vi "parse_speed.vi"(11 "Up Speed(mm/min)":dbl) -> (3 "String":string)   [LabVIEW 2017]
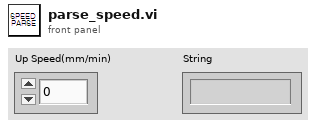
[diagram p1: front panel]
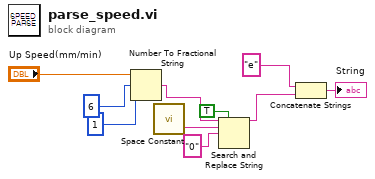
[diagram p0: block diagram]
diagram:
  n1 = Number To Fractional String(number="Up Speed(mm/min)", width (-)=6, precision (6)=1) -> (F-format string=w6:string)  [unwired: 1 in]
  n2 = call <vilib>:"Space Constant.vi"() -> ("String"=w4:string)
  n3 = Search and Replace String(replace all?=TRUE, input string=w6, search string=w4, replace string="0") -> (result string=w8:string)  [unwired: 4 in, 3 out]
  n4 = Concatenate Strings("e", w8) -> (→"String":string)
